vi "Write Value.vi"(8 "error in (no error)":errorcluster, 9 "Value":refnum<class "Scalar Type.lvclass">[](array[class]), 10 "Type":refnum<class "Scalar Type.lvclass">, 11 "fixed32 in":refnum<class "packed.lvclass">) -> (0 "error out":errorcluster, 3 "fixed32 out":refnum<class "packed.lvclass">)   [LabVIEW 2020, in "Protobuf RAW.lvlib" / "packed.lvclass"]
uses:
  packed.lvclass
  Scalar Encoder/Scalar Type.lvclass
  packed.lvclass/packed.ctl
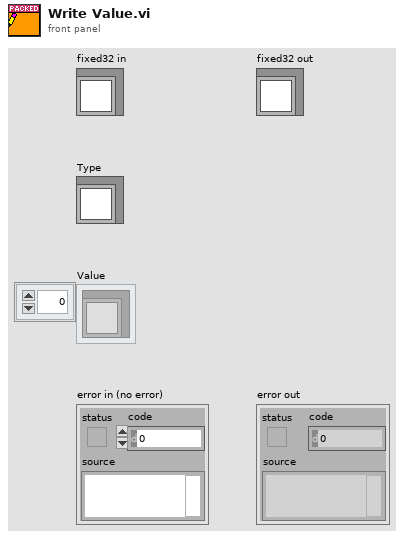
[diagram p1: front panel]
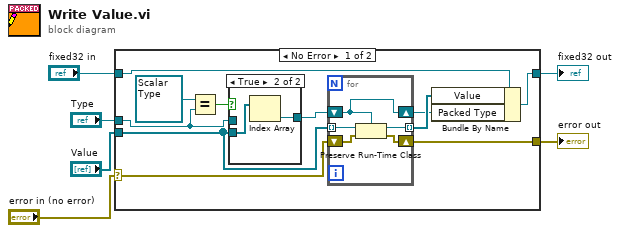
[diagram p0: block diagram]
diagram:
  n1 = case shown="No Error" "error in (no error)" {
    selector: "error in (no error)" -> [w12 w26]
    tunnel: [w10 w26] -> w5
    tunnel: [w16 w27] -> w3
    tunnel: "fixed32 in" -> [w17 w27]
    tunnel: "Value" -> [w8 _]
    tunnel: "Type" -> [w15 _]
    frame No Error {
      n2 = Equal?(x=refnum<class "Scalar Type.lvclass"> refnum ("y"), y=w15) -> (x = y?=w13:bool)
      n3 = case shown="True" w13 {
        tunnel: w15 -> [w23 _]
        tunnel: [w23 w24] -> w9
        tunnel: w8 -> [_ w25]
        frame False {
        }
        frame True {
          n4 = Index Array(array=w25) -> (element=w24:refnum<class "Scalar Type.lvclass">)  [unwired: 1 in]
        }
      }
      n5 = for {
        tunnel: w8 -> [w22] mode=indexing
        tunnel: [w21] -> w11 mode=indexing
        shift-right: [w19] -> w10
        shift-left: w12 -> [w20]
        shift-right: [w18] -> w7
        shift-left: w9 -> [w18]
        n6 = Preserve Run-Time Class(object in=w22, error in=w20, 2:w18) -> (object out=w21:refnum<class "Scalar Type.lvclass">, error out=w19:errorcluster)
      }
      n7 = Bundle By Name(cluster=w17, "Value"=w11, "Packed Type"=w7) -> (w16:refnum<class "packed.lvclass">)
    }
    frame Error {
    }
  }
  "error out" <- w5
  "fixed32 out" <- w3
